vi "Assert System Definition File Mutated.vi"(8 "error in (no error)":errorcluster, 10 "Mutated System Definition File":path, 11 "Embedded Data Logger Unit Tests in":refnum<class "Embedded Data Logger Unit Tests.lvclass">) -> (0 "error out":errorcluster, 3 "Embedded Data Logger Unit Tests out":refnum<class "Embedded Data Logger Unit Tests.lvclass">)   [LabVIEW 2027, in "Embedded Data Logger Unit Tests.lvclass"]
uses:
  Embedded Data Logger Unit Tests.lvclass
  Embedded Data Logger Unit Tests.lvclass/Embedded Data Logger Unit Tests.ctl
  C:/NetCore/niveristand-embedded-data-logger-custom-device/Source/Tests/Unit/Assert System Definition File Mutated.vi/NationalInstruments.VeriStand.SystemDefinitionAPI
  NationalInstruments.VeriStand.SystemDefinitionAPI
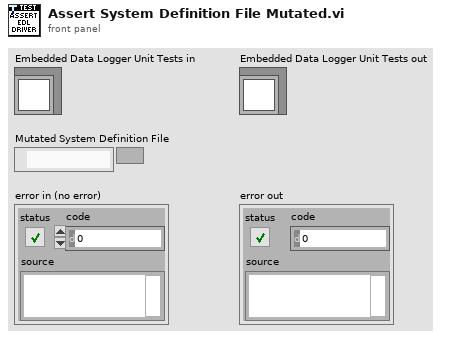
[diagram p1: front panel]
types:
  T1 = cluster{"Path":string, "RTDestination":string, "SupportedTarget":string, "Type":i32, "Version":string}[]
  T2 = cluster{"Path":string, "RTDestination":string, "SupportedTarget":string, "Type":i32, "Version":string}
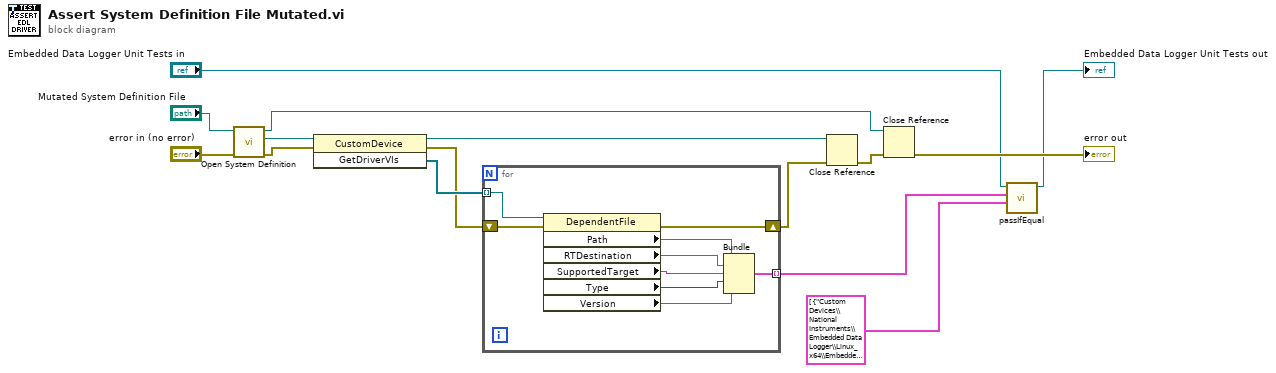
[diagram p0: block diagram]
diagram:
  n1 = call "Open System Definition.vi"("error in (no error)"="error in (no error)", "System Definition File"="Mutated System Definition File") -> ("error out"=w10:errorcluster, "NationalInstruments.VeriStand.SystemDefinitionAPI.CustomDevice"=w11:refnum<k39>, "NationalInstruments.VeriStand.SystemDefinitionAPI.SystemDefinition"=w14:refnum<k39>)  [unwired: 7 in]
  n2 = invoke class="CustomDevice" method="GetDriverVIs"(reference=w11, error in=w10) -> (reference out=w8:refnum<k39>, error out=w6:errorcluster, "GetDriverVIs"=w7:refnum<k39>[])  [unwired: 1 in]
  n3 = for {
    tunnel: w7 -> [w24] mode=indexing
    tunnel: [w18] -> w2 mode=indexing
    shift-right: [w16] -> w5
    shift-left: w6 -> [w17]
    n4 = property class="DependentFile"(reference=w24, error in=w17) -> (error out=w16:errorcluster, "Path"=w23:string, "RTDestination"=w22:string, "SupportedTarget"=w21:string, "Type"=w20:i32, "Version"=w19:string)  [unwired: 1 out]
    n5 = Bundle("Path"=w23, "RTDestination"=w22, "SupportedTarget"=w21, "Type"=w20, "Version"=w19) -> (w18:T2)  [unwired: 1 in]
  }
  n6 = Close Reference(reference=w8, error in (no error)=w5) -> (error out=w9:errorcluster)
  n7 = Close Reference(reference=w14, error in (no error)=w9) -> (error out=→"error out":errorcluster)
  n8 = call-dynamic "passIfEqual.vi"("y"=T1 [{"Path"="Custom Devices\\National Instruments\\Embedded Data Logger\\Linux_x64\\Embedded Data Logger Engine Linux64.llb\\RT Driver VI.vi", "RTDestination"="c:\\ni-rt\\NIVeriStand\\Custom Devices\\National Instruments\\Embedded Data Logger\\Embedded Data Logger Engine Linux64.llb\\RT Driver VI.vi", "SupportedTarget"="Linux_x64", "Type"=2, "Version"="2020.0.0.0"}, {"Path"="Custom Devices\\National Instruments\\Embedded Data Logger\\Linux_32_ARM\\Embedded Data Logger Engine LinuxARM.llb\\RT Driver VI.vi", "RTDestination"="c:\\ni-rt\\NIVeriStand\\Custom Devices\\National Instruments\\Embedded Data Logger\\Embedded Data Logger Engine LinuxARM.llb\\RT Driver VI.vi", "SupportedTarget"="Linux_32_ARM", "Type"=2, "Version"="2020.0.0.0"}, {"Path"="Custom Devices\\National Instruments\\Embedded Data Logger\\PharLap\\Embedded Data Logger Engine Pharlap.llb\\RT Driver VI.vi", "RTDestination"="c:\\ni-rt\\NIVeriStand\\Custom Devices\\National Instruments\\Embedded Data Logger\\Embedded Data Logger Engine Pharlap.llb\\RT Driver VI.vi", "SupportedTarget"="PharLap", "Type"=2, "Version"="2020.0.0.0"}, {"Path"="Custom Devices\\National Instruments\\Embedded Data Logger\\Windows\\Embedded Data Logger Engine Windows.llb\\RT Driver VI.vi", "RTDestination"="c:\\ni-rt\\NIVeriStand\\Custom Devices\\National Instruments\\Embedded Data Logger\\Embedded Data Logger Engine Windows.llb\\RT Driver VI.vi", "SupportedTarget"="Windows", "Type"=2, "Version"="2020.0.0.0"}] ("Array 2"), "x"=w2, "TestCase in"="Embedded Data Logger Unit Tests in") -> ("TestCase out"=→"Embedded Data Logger Unit Tests out":refnum<class "Embedded Data Logger Unit Tests.lvclass">)  [unwired: 7 in, 1 out]
